vi "FromTimeAndTemp.vi"(8 "error in (no error)":errorcluster, 9 "temperature":dbl, 10 "time":dbl, 11 "dvotTTPathPoint in":refnum<class "dvotTTPathPoint.lvclass">) -> (0 "error out":errorcluster, 3 "dvotTTPathPoint out":refnum<class "dvotTTPathPoint.lvclass">)   [LabVIEW 2012, in "dvotTTPathPoint.lvclass"]
uses:
  dvotTTPathPoint.lvclass
  dvotTTPathPoint.lvclass/dvotTTPathPoint.ctl
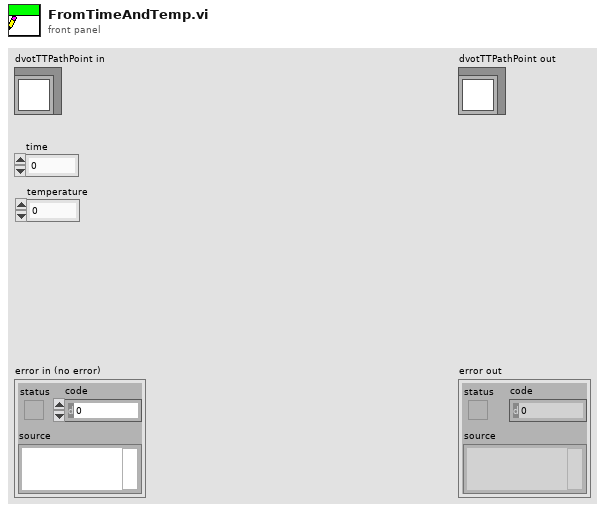
[diagram p1: front panel]
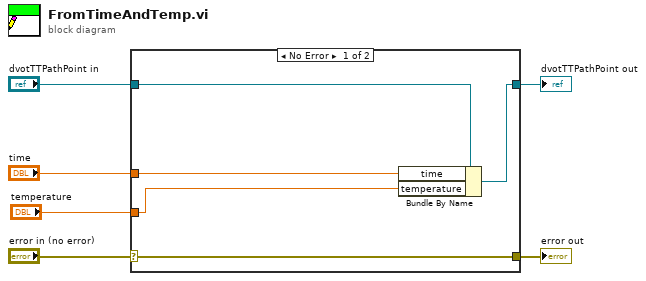
[diagram p0: block diagram]
diagram:
  n1 = case shown="No Error" "error in (no error)" {
    selector: "error in (no error)" -> [w11 w12]
    tunnel: [w11 w12] -> w5
    tunnel: [w9 w13] -> w3
    tunnel: "dvotTTPathPoint in" -> [w10 w13]
    tunnel: "time" -> [w8 _]
    tunnel: "temperature" -> [w7 _]
    frame No Error {
      n2 = Bundle By Name(cluster=w10, "time"=w8, "temperature"=w7) -> (w9:refnum<class "dvotTTPathPoint.lvclass">)
    }
    frame Error {
    }
  }
  "error out" <- w5
  "dvotTTPathPoint out" <- w3
